vi "GIF Load and Size Reader.vi"(8 "error in (no error)":errorcluster, 10 "Graphic":path, 11 "Pop-Up.lvlib:Gif Parent.lvclass":refnum<class "GIF Parent.lvclass">) -> (0 "error out":errorcluster, 1 "pic height":i16, 2 "pic width":i16, 3 "Pop-Up.lvlib:Gif Parent.lvclass out":refnum<class "GIF Parent.lvclass">, 5 "Images":T1[](array[typedef]))   [LabVIEW 2021, in "GIF Parent.lvclass"]
doc: "get the information for the size of the custom image and the background info\n\n<b>Code Developed By:</b>\nTechnology Service Corporation\n1983 S Liberty Drive\nBloomington, IN 47403\nPhone: 812 558-7100\nwww.tsc.com/atcs"
uses:
  GIF Parent.lvclass
  <vilib>/picture/picture.llb/imagedata.ctl
  GIF Parent.lvclass/GIF Parent.ctl
  <vilib>/Dataflow_G/G-Image/Image IO/Polymorphic VIs/Load Animated GIF Image (Path).vi
  <vilib>/Dataflow_G/G-Image/G-Image.lvlib
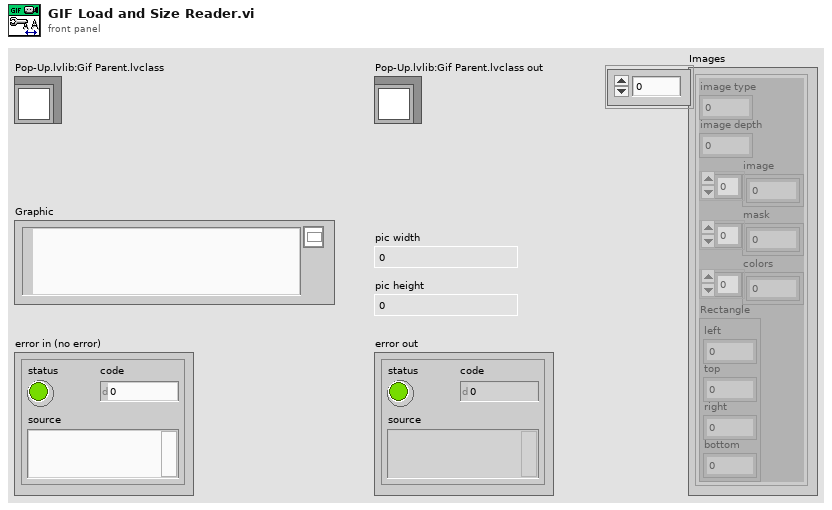
[diagram p1: front panel]
types:
  T1 = typedef "imagedata.ctl" = cluster{"image type":i32, "image depth":i32, "image":u8[], "mask":u8[], "colors":u32[], "Rectangle":cluster{"left":i16, "top":i16, "right":i16, "bottom":i16}}
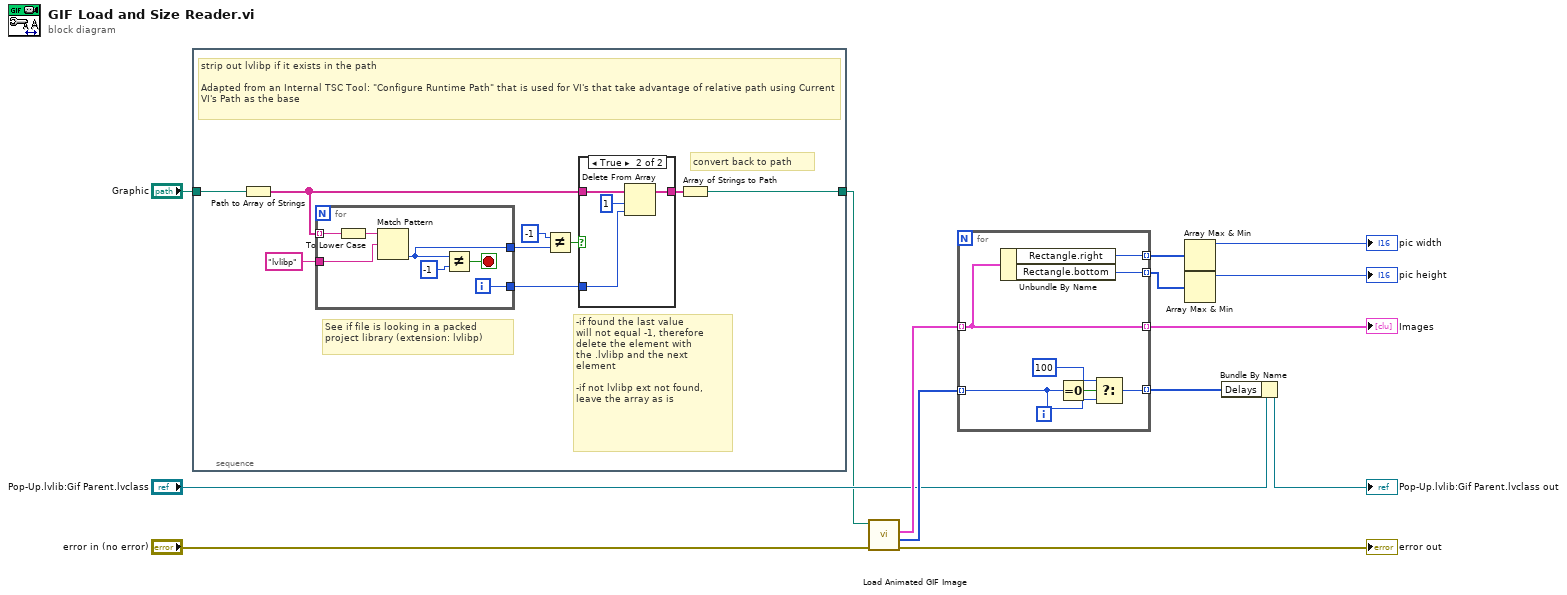
[diagram p0: block diagram]
diagram:
  n1 = stacked-sequence {
    tunnel: [w15] -> w1
    tunnel: "Graphic" -> [w16]
    frame #0 {
      # "convert back to path"
      # "-if found the last value\nwill not equal -1, therefore\ndelete the element with\nthe .lvlibp and the next\nelement\n\n-if not lvlibp ext not found,\nleave the array as is"
      # "See if file is looking in a packed\nproject library (extension: lvlibp)"
      # "strip out lvlibp if it exists in the path\n\nAdapted from an Internal TSC Tool: \"Configure Runtime Path\" that is used for VI's that take advantage of relative path using Current VI's Path as the base"
      n2 = Path to Array of Strings(0:w16) -> (2:w22:string[])  [unwired: 1 out]
      n3 = for {
        tunnel: w22 -> [w35] mode=indexing
        tunnel: "lvlibp" ("element") -> [w33]
        tunnel: [w32] -> w21
        tunnel: [w29] -> w20
        i -> [w32]
        stop <- w30 stop-if-true
        n4 = To Lower Case(string=w35) -> (all lower case string=w34:string)
        n5 = Match Pattern(string=w34, regular expression=w33) -> (offset past match=w29:i32)  [unwired: 1 in, 3 out]
        n6 = Not Equal?(x=w29, y=-1) -> (x != y?=w30:bool)
      }
      n7 = Not Equal?(x=-1 ("y"), y=w20) -> (x != y?=w18:bool)
      n8 = case shown="True" w18 {
        tunnel: w22 -> [w24 w28]
        tunnel: w21 -> [_ w27]
        tunnel: [w24 w25] -> w17
        frame False {
        }
        frame True {
          n9 = Delete From Array(array=w28, length=1, index=w27) -> (array with subset deleted=w25:string[])  [unwired: 1 out]
        }
      }
      n10 = Array of Strings to Path(0:w17) -> (2:w15:path)  [unwired: 1 in]
    }
  }
  n11 = call-poly <vilib>:"Load Animated GIF Image.vi"("error in (no error)"="error in (no error)", "Path In"=w1) -> ("error out"=→"error out":errorcluster, "Delays"=w11:i32[], "Frames"=w12:T1[])  [unwired: 6 in, 1 out]
  n12 = for {
    tunnel: w11 -> [w40] mode=indexing
    tunnel: [w39] -> w4 mode=indexing
    tunnel: w12 -> [w38] mode=indexing
    tunnel: [w38] -> w3 mode=indexing
    tunnel: [w37] -> w10 mode=indexing
    tunnel: [w36] -> w8 mode=indexing
    n13 = Unbundle By Name(w38) -> ("Rectangle.right"=w36:i16, "Rectangle.bottom"=w37:i16)
    n14 = Equal To 0?(x=w40) -> (x = 0?=w42:bool)
    n15 = Select(t=100, s=w42, f=w40) -> (s? t:f=w39:i32)
  }
  "Images" <- w3
  n16 = Array Max & Min(array=w8) -> (max value=→"pic width":i16)  [unwired: 3 out]
  n17 = Array Max & Min(array=w10) -> (max value=→"pic height":i16)  [unwired: 3 out]
  n18 = Bundle By Name(cluster="Pop-Up.lvlib:Gif Parent.lvclass", "Delays"=w4) -> (→"Pop-Up.lvlib:Gif Parent.lvclass out":refnum<class "GIF Parent.lvclass">)
